vi "Init Temp Controller.vi"(8 "error in (no error)":errorcluster, 11 "Application in":refnum<class "Application.lvclass">) -> (0 "error out":errorcluster, 3 "Application out":refnum<class "Application.lvclass">)   [LabVIEW 2023, in "Application.lvlib" / "Application.lvclass"]
uses:
  Application.lvclass
  C:/Program Files/National Instruments/LabVIEW 2023/vi.lib/ActorFramework/Actor/Actor.lvclass
  Hardware/Temperature Controller/Temperature Controller.lvclass
  Application.lvclass/Application.ctl
  User Interface/Splash Screen Messages/Update Status Msg/Update Status Msg.lvclass/Update Status Msg.ctl
  <vilib>/ActorFramework/Message Enqueuer/Message Enqueuer.lvclass/Message Enqueuer.ctl
  <vilib>/ActorFramework/Message Enqueuer/Enqueue.vi
  User Interface/Splash Screen Messages/Update Status Msg/Update Status Msg.lvclass
  C:/Program Files/National Instruments/LabVIEW 2023/vi.lib/ActorFramework/Message/Message.lvclass
  <vilib>/ActorFramework/Message Priority Queue/Priority Enqueue.vi
  <vilib>/ActorFramework/Actor/Actor.lvclass
  C:/FLASH/Development/Hardware/Device/Device.lvclass
  C:/FLASH/Development/Hardware/Temperature Controller/Temperature Controller.lvclass
  C:/FLASH/Development/Application/Application.lvclass
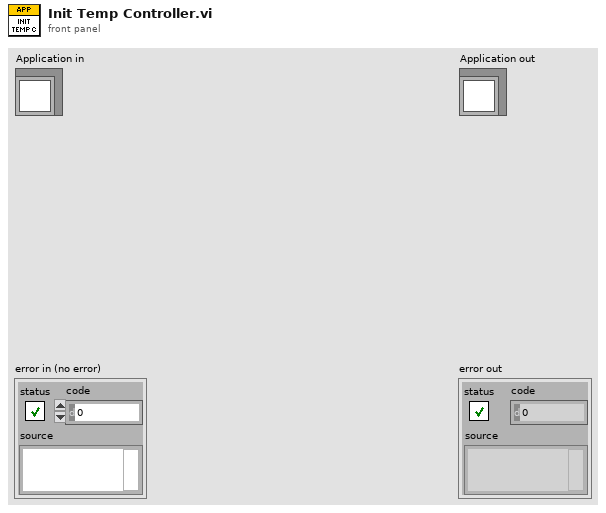
[diagram p1: front panel]
types:
  T1 = typedef "Temp Controller Configuration.ctl" = cluster{"COM Port":refnum<visa-resource-name>, "Type":enum16{"Disabled", "TC-720"}}
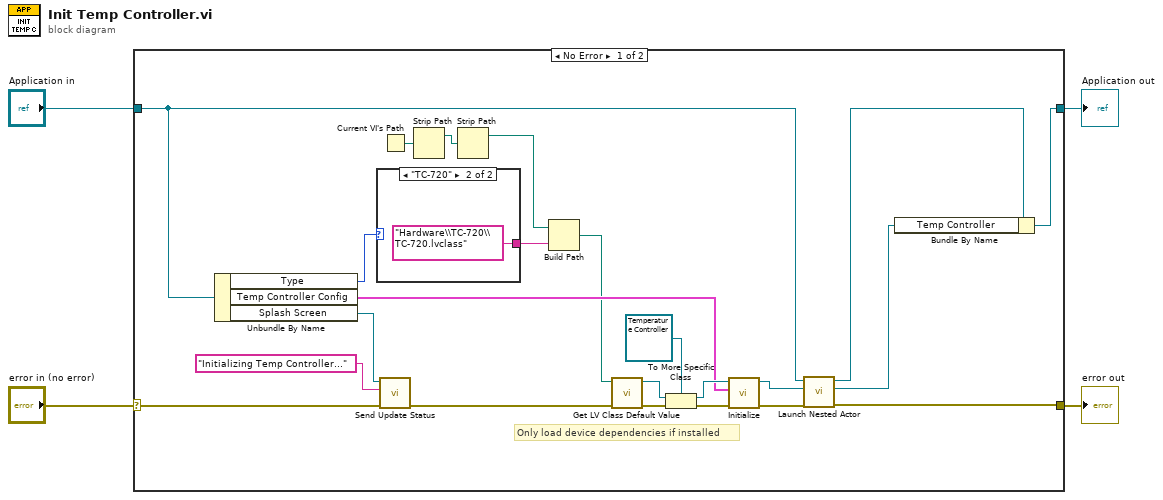
[diagram p0: block diagram]
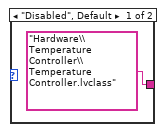
[diagram p2: hidden frame]
diagram:
  n1 = case shown="No Error" "error in (no error)" {
    selector: "error in (no error)" -> [w26 w31]
    tunnel: [w23 w31] -> w3
    tunnel: [w19 w30] -> w1
    tunnel: "Application in" -> [w21 w30]
    frame No Error {
      # "Only load device dependencies if installed"
      n2 = Unbundle By Name(w21) -> ("Type"=w7:enum16{"Disabled", "TC-720"}, "Temp Controller Config"=w11:T1, "Splash Screen"=w25:refnum<class "Message Enqueuer.lvclass">)
      n3 = case shown="\"TC-720\"" w7 {
        tunnel: ["Hardware\\Temperature Controller\\Temperature Controller.lvclass" "Hardware\\TC-720\\TC-720.lvclass"] -> w6
        frame "Disabled", Default {
        }
        frame "TC-720" {
        }
      }
      n4 = call "Send Update Status.vi"("error in (no error)"=w26, "Status Message"="Initializing Temp Controller...", "Message Enqueuer"=w25) -> ("error out"=w16:errorcluster)  [unwired: 7 in, 1 out]
      n5 = Current VI's Path() -> (path=w10:path)
      n6 = Strip Path(path=w10) -> (stripped path=w9:path)  [unwired: 1 out]
      n7 = Strip Path(path=w9) -> (stripped path=w8:path)  [unwired: 1 out]
      n8 = Build Path(base path=w8, name or relative path=w6) -> (appended path=w5:path)
      n9 = call <vilib>:"Get LV Class Default Value.vi"("error in (no error)"=w16, "class path"=w5) -> ("error out"=w17:errorcluster, "object"=w13:refnum<class>)  [unwired: 8 in]
      n10 = To More Specific Class(target class=refnum<class "Temperature Controller.lvclass"> refnum ("Temperature Controller.lvlib:Temperature Controller.lvclass"), reference=w13, error in=w17) -> (specific class reference=w12:refnum<class "Temperature Controller.lvclass">, error out=w15:errorcluster)
      n11 = call-dynamic "Initialize.vi"("error in (no error)"=w15, "Temp Conotroller Config"=w11, "Temperature Controller in"=w12) -> ("error out"=w24:errorcluster, "Temperature Controller out"=w22:refnum<class "Temperature Controller.lvclass">)  [unwired: 7 in]
      n12 = call <vilib>:"Launch Nested Actor.vi"("error in (no error)"=w24, "Nested Actor"=w22, "Caller Actor in"=w21) -> ("error out"=w23:errorcluster, "Nested Actor's Enqueuer"=w18:refnum<class "Message Enqueuer.lvclass">, "Caller Actor out"=w20:refnum<class "Application.lvclass">)  [unwired: 6 in]
      n13 = Bundle By Name(cluster=w20, "Temp Controller"=w18) -> (w19:refnum<class "Application.lvclass">)
    }
    frame Error {
    }
  }
  "error out" <- w3
  "Application out" <- w1
